vi "Save_Data_In_TDMS.vi"(7 "tdms file":refnum<k34>, 10 "Save Data":bool, 11 "data":dbl[](array[numeric])) -> (0 "error out":errorcluster, 3 "tdms file out":refnum<k34>)   [LabVIEW 2019]
panel:
  out "channel name(s) in (Untitled)":string[](array[string])=["MainLoopTime [ms]", "AppliedForceTranslation [N]", "AppliedTorqueRotation [Nmm]", "RelPosTrans [mm]", "AbsPosTrans [mm]", "VelTrans [mm/s]", "RelPosRot [°]", "AbsPosRot [°]", "VelRot [°/s]", "MotorModeRot", "StopPosRot [°]", "MovePosRot [°]", "MoveVelRot [°/s]", "StartPosRot1 [°]", "MiddlePosRot1 [°]", "EndPosRot1 [°]", "ForceConstRot1", "isDamperRot1", "StartPosRot2 [°]", "MiddlePosRot2 [°]", "EndPosRot2 [°]", "ForceConstRot2 ", "isDamperRot2", "StartPosRot3 [°]", "MiddlePosRot3 [°]", "EndPosRot3 [°]", "ForceConstRot3", "isDamperRot3", "StartPosRot4 [°]", "MiddlePosRot4 [°]", "EndPosRot4 [°]", "ForceConstRot4 ", "isDamperRot4", "StartPosRot5 [°]", "MiddlePosRot5 [°]", "EndPosRot5 [°]", "ForceConstRot5", "isDamperRot5", "StartPosRot6 [°]", "MiddlePosRot6 [°]", "EndPosRot6 [°]", "ForceConstRot6", "isDamperRot6", "StartPosRot7 [°]", "MiddlePosRot7 [°]", "EndPosRot7 [°]", "ForceConstRot7", "isDamperRot7", "StartPosRot8 [°]", "MiddlePosRot8 [°]", "EndPosRot8 [°]", "ForceConstRot8", "isDamperRot8", "StartPosRot9 [°]", "MiddlePosRot9 [°]", "EndPosRot9 [°]", "ForceConstRot9", "isDamperRot9", "StartPosRot10 [°]", "MiddlePosRot10 [°]", "EndPosRot10 [°]", "ForceConstRot10", "isDamperRot10", "PertAmpRot [°]", "PertTimeRot [ms]", "PertSignRot", "PertTgtPosRot [°]", "DeltaOSRot [Nmm]", "BaselineOSRot [Nmm]", "DeltaOFRot [Nmm]", "BaselineOFRot [Nmm]", "DeltaCSRot [Nmm]", "BaselineCSRot [Nmm]", "DeltaCFRot [Nmm]", "BaselineCFRot [Nmm]", "MotorModeTrans", "StopPosTrans [mm]", "MovePosTrans [mm]", "MoveVelTrans [mm/s]", "StartPosTrans1 [mm]", "MiddlePosTrans1 [mm]", "EndPosTrans1 [mm]", "ForceConstTrans1", "isDamperTrans1", "StartPosTrans2 [mm]", "MiddlePosTrans2 [mm]", "EndPosTrans2 [mm]", "ForceConstTrans2", "isDamperTrans2", "StartPosTrans3 [mm]", "MiddlePosTrans3 [mm]", "EndPosTrans3 [mm]", "ForceConstTrans3", "isDamperTrans3", "StartPosTrans4 [mm]", "MiddlePosTrans4 [mm]", "EndPosTrans4 [mm]", "ForceConstTrans4", "isDamperTrans4", "StartPosTrans5 [mm]", "MiddlePosTrans5 [mm]", "EndPosTrans5 [mm]", "ForceConstTrans5", "isDamperTrans5", "StartPosTrans6 [mm]", "MiddlePosTrans6 [mm]", "EndPosTrans6 [mm]", "ForceConstTrans6", "isDamperTrans6", "StartPosTrans7 [mm]", "MiddlePosTrans7 [mm]", "EndPosTrans7 [mm]", "ForceConstTrans7", "isDamperTrans7", "StartPosTrans8 [mm]", "MiddlePosTrans8 [mm]", "EndPosTrans8 [mm]", "ForceConstTrans8", "isDamperTrans8", "StartPosTrans9 [mm]", "MiddlePosTrans9 [mm]", "EndPosTrans9 [mm]", "ForceConstTrans9", "isDamperTrans9", "StartPosTrans10 [mm]", "MiddlePosTrans10 [mm]", "EndPosTrans10 [mm]", "ForceConstTrans10", "isDamperTrans10", "PertAmpTrans [mm]", "PertTimeTrans [ms]", "PertSignTrans", "PertTgtPosTrans [mm]", "DeltaOSTrans [N]", "BaselineOSTrans [N]", "DeltaOFTrans [N]", "BaselineOFTrans [N]", "DeltaCSTrans [N]", "BaselineCSTrans [N]", "DeltaCFTrans [N]", "BaselineCFTrans [N]", "Mode", "GameMode", "Level", "CorrectAnswers", "TotalAnswers", "Repetitions", "SoftSafety", "HardSafety", "PotiPosRot [°]", "PotiPosTrans [mm]", "RightPotiTransVolt [V]", "LeftPotiTransVolt [V]"]
  # "This Vi saves the exercise data and settings in a TDMS file."
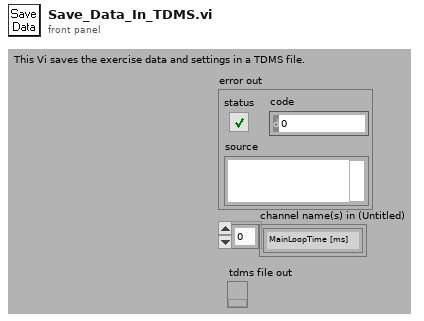
[diagram p1: front panel]
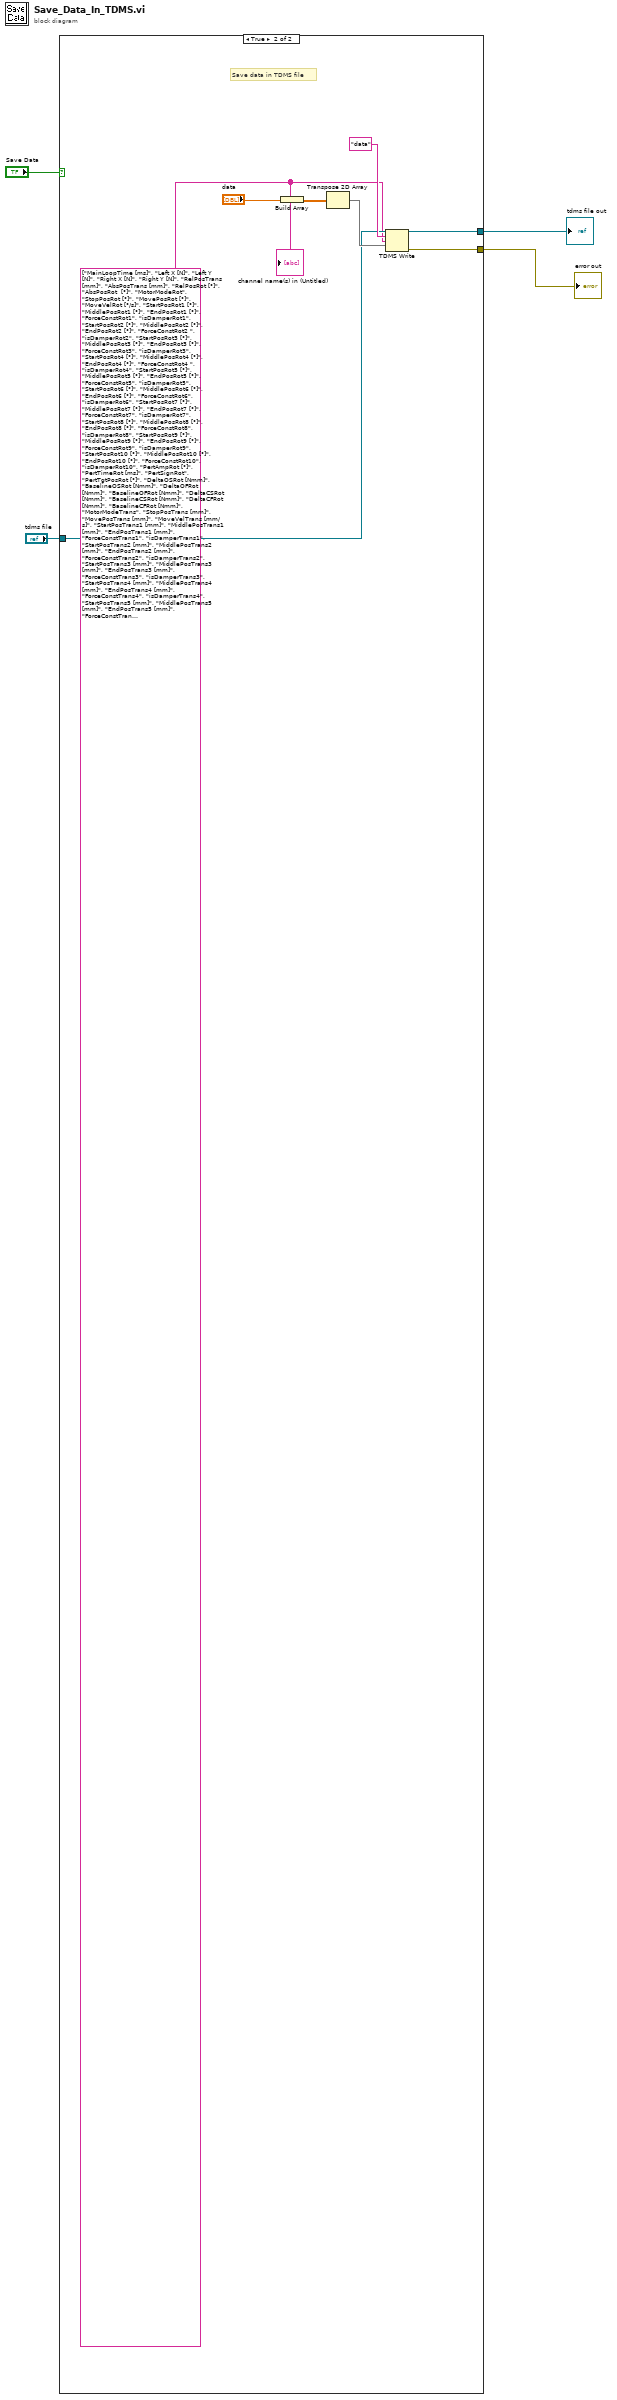
[diagram p0: block diagram]
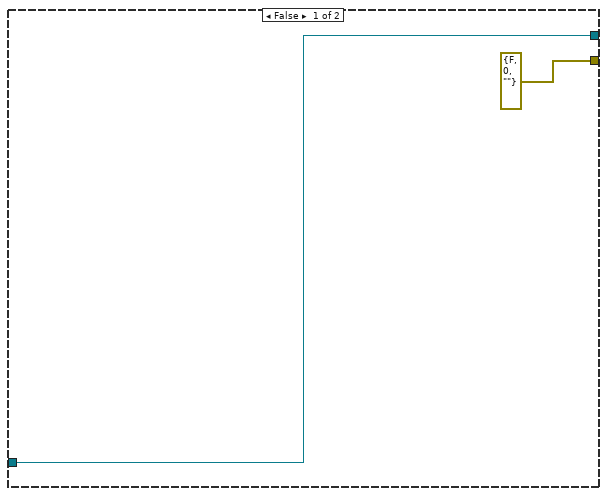
[diagram p2: hidden frame]
diagram:
  n1 = case shown="True" "Save Data" {
    tunnel: [w6 w10] -> w2
    tunnel: "tdms file" -> [w6 w9]
    tunnel: [errorcluster {"status"=FALSE, "code"=0, "source"=""} ("error out") w7] -> w1
    frame False {
    }
    frame True {
      w8 = string[] ["MainLoopTime [ms]", "Left X [N]", "Left Y [N]", "Right X [N]", "Right Y [N]", "RelPosTrans [mm]", "AbsPosTrans [mm]", "RelPosRot [°]", "AbsPosRot  [°]", "MotorModeRot", "StopPosRot [°]", "MovePosRot [°]", "MoveVelRot [°/s]", "StartPosRot1 [°]", "MiddlePosRot1 [°]", "EndPosRot1 [°]", "ForceConstRot1", "isDamperRot1", "StartPosRot2 [°]", "MiddlePosRot2 [°]", "EndPosRot2 [°]", "ForceConstRot2 ", "isDamperRot2", "StartPosRot3 [°]", "MiddlePosRot3 [°]", "EndPosRot3 [°]", "ForceConstRot3", "isDamperRot3", "StartPosRot4 [°]", "MiddlePosRot4 [°]", "EndPosRot4 [°]", "ForceConstRot4 ", "isDamperRot4", "StartPosRot5 [°]", "MiddlePosRot5 [°]", "EndPosRot5 [°]", "ForceConstRot5", "isDamperRot5", "StartPosRot6 [°]", "MiddlePosRot6 [°]", "EndPosRot6 [°]", "ForceConstRot6", "isDamperRot6", "StartPosRot7 [°]", "MiddlePosRot7 [°]", "EndPosRot7 [°]", "ForceConstRot7", "isDamperRot7", "StartPosRot8 [°]", "MiddlePosRot8 [°]", "EndPosRot8 [°]", "ForceConstRot8", "isDamperRot8", "StartPosRot9 [°]", "MiddlePosRot9 [°]", "EndPosRot9 [°]", "ForceConstRot9", "isDamperRot9", "StartPosRot10 [°]", "MiddlePosRot10 [°]", "EndPosRot10 [°]", "ForceConstRot10", "isDamperRot10", "PertAmpRot [°]", "PertTimeRot [ms]", "PertSignRot", "PertTgtPosRot [°]", "DeltaOSRot [Nmm]", "BaselineOSRot [Nmm]", "DeltaOFRot [Nmm]", "BaselineOFRot [Nmm]", "DeltaCSRot [Nmm]", "BaselineCSRot [Nmm]", "DeltaCFRot [Nmm]", "BaselineCFRot [Nmm]", "MotorModeTrans", "StopPosTrans [mm]", "MovePosTrans [mm]", "MoveVelTrans [mm/s]", "StartPosTrans1 [mm]", "MiddlePosTrans1 [mm]", "EndPosTrans1 [mm]", "ForceConstTrans1", "isDamperTrans1", "StartPosTrans2 [mm]", "MiddlePosTrans2 [mm]", "EndPosTrans2 [mm]", "ForceConstTrans2", "isDamperTrans2", "StartPosTrans3 [mm]", "MiddlePosTrans3 [mm]", "EndPosTrans3 [mm]", "ForceConstTrans3", "isDamperTrans3", "StartPosTrans4 [mm]", "MiddlePosTrans4 [mm]", "EndPosTrans4 [mm]", "ForceConstTrans4", "isDamperTrans4", "StartPosTrans5 [mm]", "MiddlePosTrans5 [mm]", "EndPosTrans5 [mm]", "ForceConstTrans5", "isDamperTrans5", "StartPosTrans6 [mm]", "MiddlePosTrans6 [mm]", "EndPosTrans6 [mm]", "ForceConstTrans6", "isDamperTrans6", "StartPosTrans7 [mm]", "MiddlePosTrans7 [mm]", "EndPosTrans7 [mm]", "ForceConstTrans7", "isDamperTrans7", "StartPosTrans8 [mm]", "MiddlePosTrans8 [mm]", "EndPosTrans8 [mm]", "ForceConstTrans8", "isDamperTrans8", "StartPosTrans9 [mm]", "MiddlePosTrans9 [mm]", "EndPosTrans9 [mm]", "ForceConstTrans9", "isDamperTrans9", "StartPosTrans10 [mm]", "MiddlePosTrans10 [mm]", "EndPosTrans10 [mm]", "ForceConstTrans10", "isDamperTrans10", "PertAmpTrans [mm]", "PertTimeTrans [ms]", "PertSignTrans", "PertTgtPosTrans [mm]", "DeltaOSTrans [N]", "BaselineOSTrans [N]", "DeltaOFTrans [N]", "BaselineOFTrans [N]", "DeltaCSTrans [N]", "BaselineCSTrans [N]", "DeltaCFTrans [N]", "BaselineCFTrans [N]", "Mode", "GameMode", "Level", "CorrectAnswers", "TotalAnswers", "Repetitions", "SoftSafety", "HardSafety", "RightPotiTransVolt [V]", "LeftPotiTransVolt [V]", "RotPotVolt [V]"] ("channel name(s) in (Untitled)")
      # "Save data in TDMS file"
      n2 = Build Array("data") -> (w12:dbl[][])
      n3 = Transpose 2D Array(2D array=w12) -> (transposed array=w13:dbl[][])
      n4 = TDMS Write(0:w9, 5:"data" ("group name in (Untitled)"), 7:w8, 9:w13) -> (4:w10:refnum<k34>, 15:w7:errorcluster)  [unwired: 2 in, 2 out]
      "channel name(s) in (Untitled)" <- w8
    }
  }
  "tdms file out" <- w2
  "error out" <- w1
